vi "Init Position_RVDT_AI Channel.vi"(8 "error in":errorcluster, 9 "Position_RVDT_Properties":T1={"Minimum Value"=-0.1, "Maximum Value"=0.1, "Excitation Source"=10200, "Excitation Wire Mode"=4, "Excitation Frequency"=2500.0, "Excitation Value"=1.0, "Units"=10146, "Sensitivity"=50.0, "Sensitivity Units"=12507, "Excitation Sense"=16095} {"Sensitivity Units" items=["mVolts/Volt/Degree"=12507, "mVolts/Volt/Radian"=12508]; "Units" items=["Degrees"=10146, "Radians"=10273, "From Custom Scale"=10065]; "Excitation Sense" items=["Local"=16095, "Remote"=16096]; "Excitation Source" items=["Internal"=10200, "External"=10167, "None"=10230]; "Excitation Wire Mode" items=["4-Wire"=4, "5-Wire"=5, "6-Wire"=6]}, 10 "physical channels":tag, 11 "task in":refnum<k21>) -> (0 "error out":errorcluster, 3 "task out":refnum<k21>)   [LabVIEW 2020, in "NI PXIe-4340 Engine.lvlib"]
uses:
  NI PXIe-4340 Engine.lvlib
  Shared/Position_RVDT_Properties.ctl
  <vilib>/DAQmx/create/channels.llb/DAQmx Create Channel (AI-Position-RVDT).vi
  <resource>/objmgr/daqmx.rc
  Shared/NI PXIe-4340 Shared.lvlib
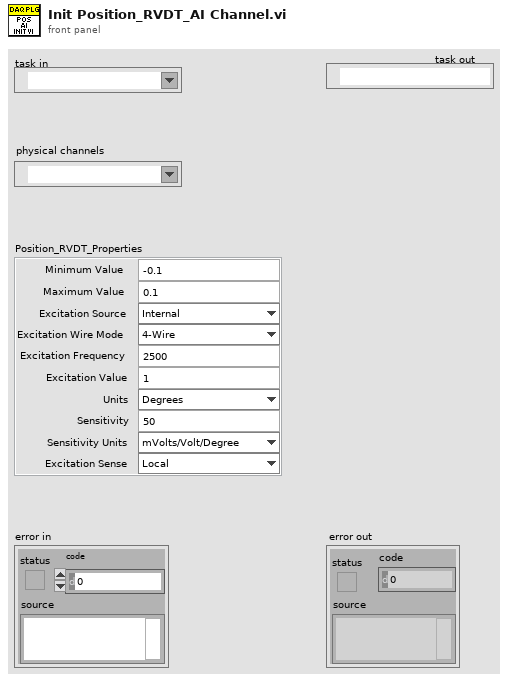
[diagram p1: front panel]
types:
  T1 = typedef "NI PXIe-4340 Shared.lvlib/Position_RVDT_Properties.ctl" = cluster{"Minimum Value":dbl, "Maximum Value":dbl, "Excitation Source":i32, "Excitation Wire Mode":i32, "Excitation Frequency":dbl, "Excitation Value":dbl, "Units":i32, "Sensitivity":dbl, "Sensitivity Units":i32, "Excitation Sense":i32}
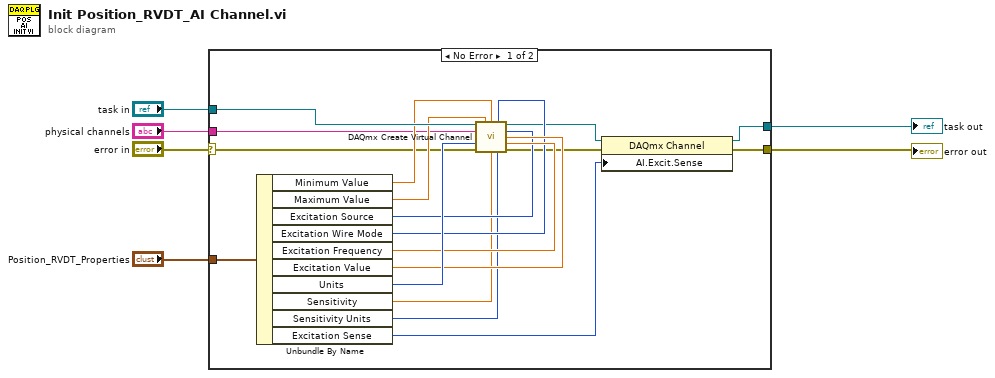
[diagram p0: block diagram]
diagram:
  n1 = case shown="No Error" "error in" {
    selector: "error in" -> [w7 w26]
    tunnel: [w13 w25] -> w6
    tunnel: [w11 w26] -> w2
    tunnel: "task in" -> [w24 w25]
    tunnel: "physical channels" -> [w21 _]
    tunnel: "Position_RVDT_Properties" -> [w8 _]
    frame No Error {
      n2 = Unbundle By Name(w8) -> ("Minimum Value"=w22:dbl, "Maximum Value"=w23:dbl, "Excitation Source"=w17:i32, "Excitation Wire Mode"=w16:i32, "Excitation Frequency"=w18:dbl, "Excitation Value"=w19:dbl, "Units"=w20:i32, "Sensitivity"=w15:dbl, "Sensitivity Units"=w14:i32, "Excitation Sense"=w9:i32)
      n3 = call-poly <vilib>:"DAQmx Create Virtual Channel.vi"("task in"=w24, "maximum value"=w23, "minimum value"=w22, "voltage excitation wire mode"=w16, "physical channels"=w21, "voltage excitation source"=w17, "voltage excitation value"=w19, "units"=w20, "voltage excitation frequency"=w18, "error in"=w7, "sensitivity"=w15, "sensitivity units"=w14) -> ("task out"=w10:refnum<k21>, "error out"=w12:errorcluster)  [unwired: 2 in]
      n4 = property class="DAQmx Channel"(reference=w10, error in=w12, "AI.Excit.Sense"=w9) -> (reference out=w13:refnum<k21>, error out=w11:errorcluster)
    }
    frame Error {
    }
  }
  "task out" <- w6
  "error out" <- w2
